vi "step_stage.vi"(4 "axis":u32, 5 "step":dbl, 6 "handle":i32, 7 "position":dbl, 8 "error in":errorcluster, 10 "+/-":bool, 11 "move":bool) -> (0 "error out":errorcluster, 1 "handle out":i32)   [LabVIEW 2019]
uses:
  Madlib.dll
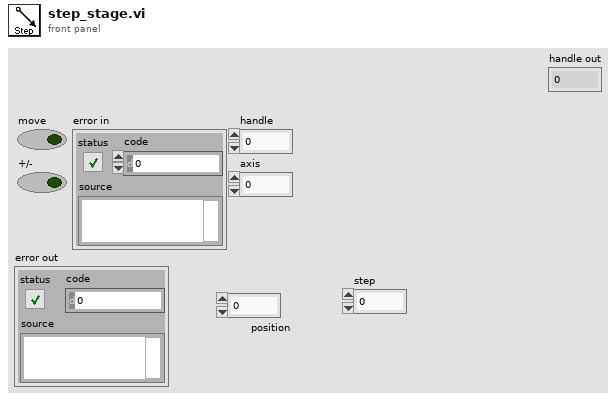
[diagram p1: front panel]
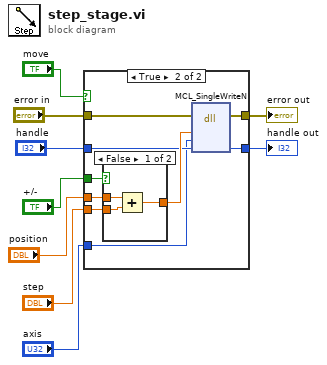
[diagram p0: block diagram]
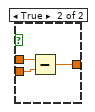
[diagram p3: hidden frame]
diagram:
  n1 = case shown="True" "move" {
    tunnel: "+/-" -> [_ w20]
    tunnel: "error in" -> [w11 w17]
    tunnel: [w11 w18] -> w4
    tunnel: "step" -> [_ w16]
    tunnel: "position" -> [_ w15]
    tunnel: "handle" -> [w10 w14]
    tunnel: "axis" -> [_ w13]
    tunnel: [w10 w12] -> w1
    frame False {
    }
    frame True {
      n2 = case shown="False" w20 {
        tunnel: w15 -> [w23 w25]
        tunnel: [w22 w26] -> w19
        tunnel: w16 -> [w21 w24]
        frame False {
          n3 = Add(x=w23, y=w21) -> (x+y=w22:dbl)
        }
        frame True {
          n4 = Subtract(x=w25, y=w24) -> (x-y=w26:dbl)
        }
      }
      n5 = dll-call lib="C:/Users/localadmin/Desktop/Ole/Nanostage/MADLib.dll" fn="MCL_SingleWriteN"(error in=w17, "position"=w19, "axis"=w13, "handle"=w14) -> (error out=w18:errorcluster, "handle"=w12:i32)  [unwired: 5 in, 1 out]
    }
  }
  "error out" <- w4
  "handle out" <- w1
